vi "DPT TC Panel Setup.vi"() -> (6 "Channel List":string="1001,1002,1003", 8 "Label Array":string[](array[string])=["RDB F", "Room Ambient(F)", "Tscale"], 10 "Indexes used":i32[](array[numeric]))   [LabVIEW 2016]
doc: "Allow user to choose TCs to measure and save data for."
uses:
  Type Definitions/DPT Channel Label.ctl
  Utility/Custom Pallet Controls/Custom Pallet String.ctl
  <vilib>/Utility/file.llb/Read From Spreadsheet File (string).vi
  <vilib>/Utility/file.llb/Write To Spreadsheet File (string).vi
panel:
  out "all rows":string[][](array[string])
  out "error out":errorcluster={"status"=TRUE, "code"=1, "source"="Set Permissions in Panel DPT Channel Test Labels.vi<APPEND>\n<Not A Path>"}
  in  "TC Panel 4":T1[][](array[typedef])
  in  "Read":bool
  in  "Write":bool
  in  "Initialize":bool
  in  "Complete":bool
  in  "TC Panel 3":T1[][](array[typedef])
  in  "TC Panel 2":T1[][](array[typedef])
  in  "TC Panel 1":T1[][](array[typedef])=[[{"Label"="RDB F", "Record"=TRUE, "Index"=0, "Channel"=""}, {"Label"="Room Ambient(F)", "Record"=TRUE, "Index"=0, "Channel"=""}, {"Label"="Tscale", "Record"=TRUE, "Index"=0, "Channel"=""}, {"Label"="", "Record"=FALSE, "Index"=0, "Channel"=""}, {"Label"="", "Record"=FALSE, "Index"=0, "Channel"=""}, {"Label"="", "Record"=FALSE, "Index"=0, "Channel"=""}], [{"Label"="", "Record"=FALSE, "Index"=0, "Channel"=""}, {"Label"="", "Record"=FALSE, "Index"=0, "Channel"=""}, {"Label"="", "Record"=FALSE, "Index"=0, "Channel"=""}, {"Label"="", "Record"=FALSE, "Index"=0, "Channel"=""}, {"Label"="", "Record"=FALSE, "Index"=0, "Channel"=""}, {"Label"="", "Record"=FALSE, "Index"=0, "Channel"=""}], [{"Label"="", "Record"=FALSE, "Index"=0, "Channel"=""}, {"Label"="", "Record"=FALSE, "Index"=0, "Channel"=""}, {"Label"="", "Record"=FALSE, "Index"=0, "Channel"=""}, {"Label"="", "Record"=FALSE, "Index"=0, "Channel"=""}, {"Label"="", "Record"=FALSE, "Index"=0, "Channel"=""}, {"Label"="", "Record"=FALSE, "Index"=0, "Channel"=""}]]
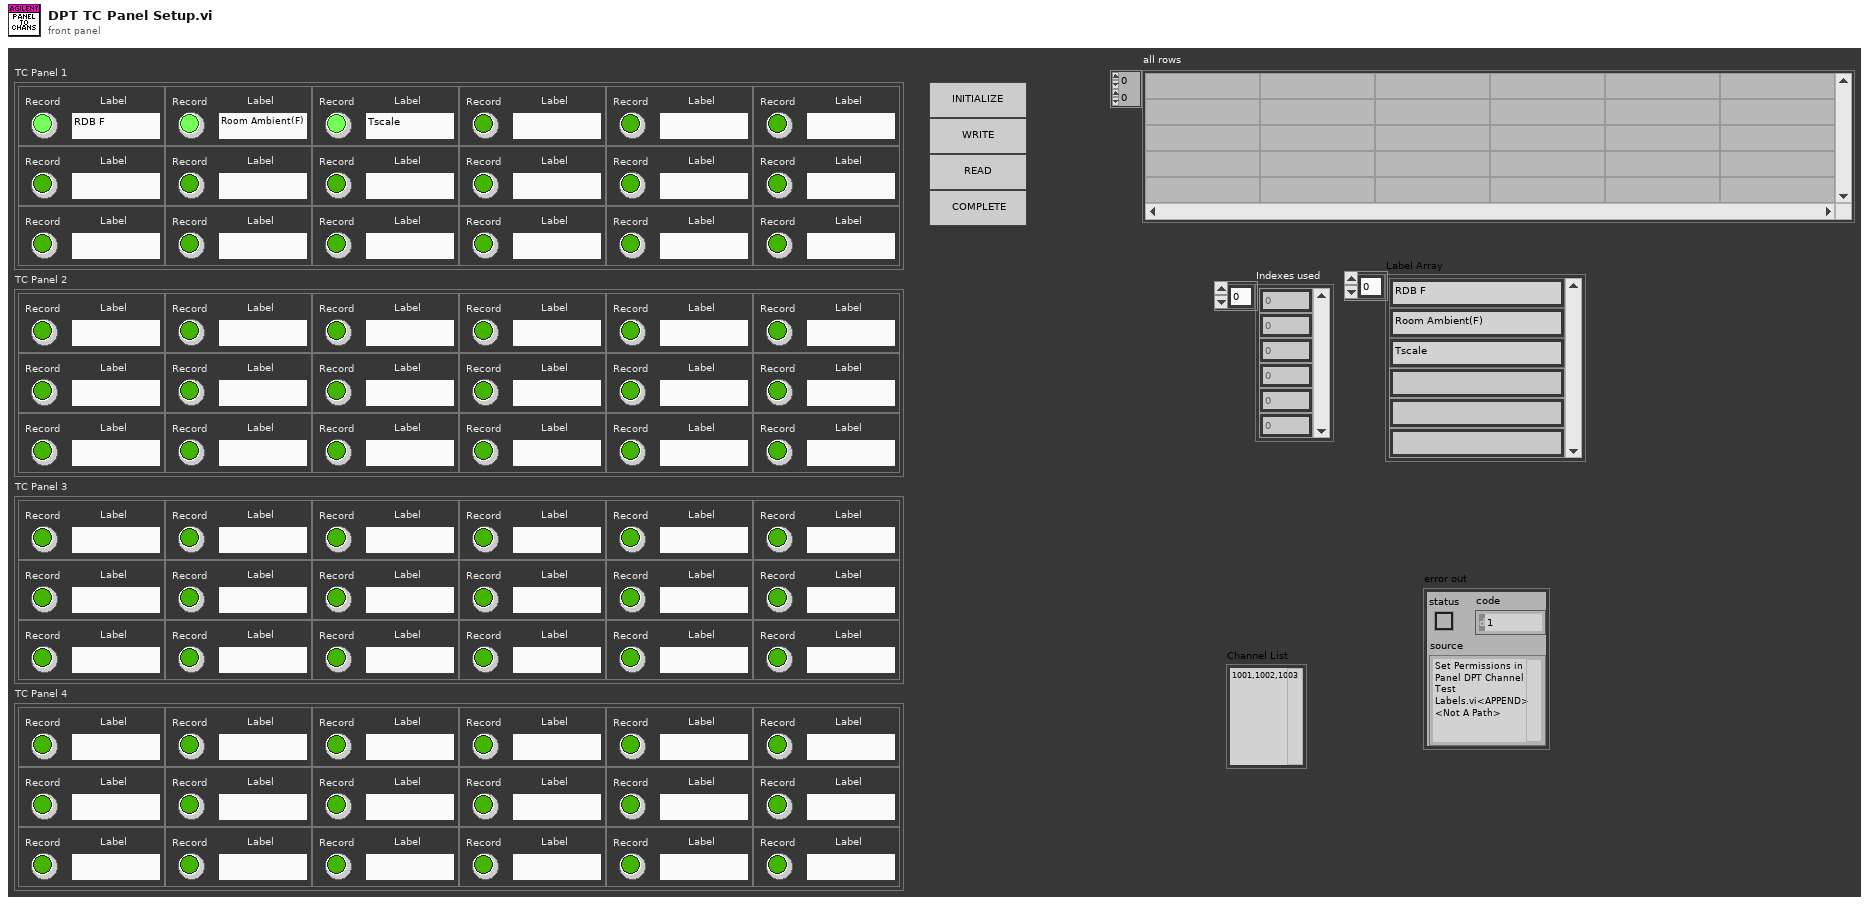
[diagram p1: front panel]
types:
  T1 = typedef "DPT Channel Label.ctl" = cluster{"Label":T2, "Record":bool, "Index":u32, "Channel":string}
  T2 = typedef "Custom Pallet String.ctl" = string
  T3 = enum32{"invalid app kind", "Development System", "Run Time System", "Student Edition", "Embedded LabVIEW", "Evaluation", "Custom"}
  T4 = enum32{"Invalid", "Standard", "Closed", "Hidden", "Minimized", "Maximized"}
  T5 = cluster{"Core":cluster{"Current VI Reference":refnum<vi>, "Close Panel on Exit?":bool}, "Array":string[][], "cDAQ index array":i32[][], "TC Panel 1":T1[][], "TC Panel 2":T1[][], "TC Panel 3":T1[][], "TC Panel 4":T1[][], "Label array":string[], "Channel array":string, "Indexes used":i32[]}
  T6 = cluster{"Current VI Reference":refnum<vi>, "Close Panel on Exit?":bool}
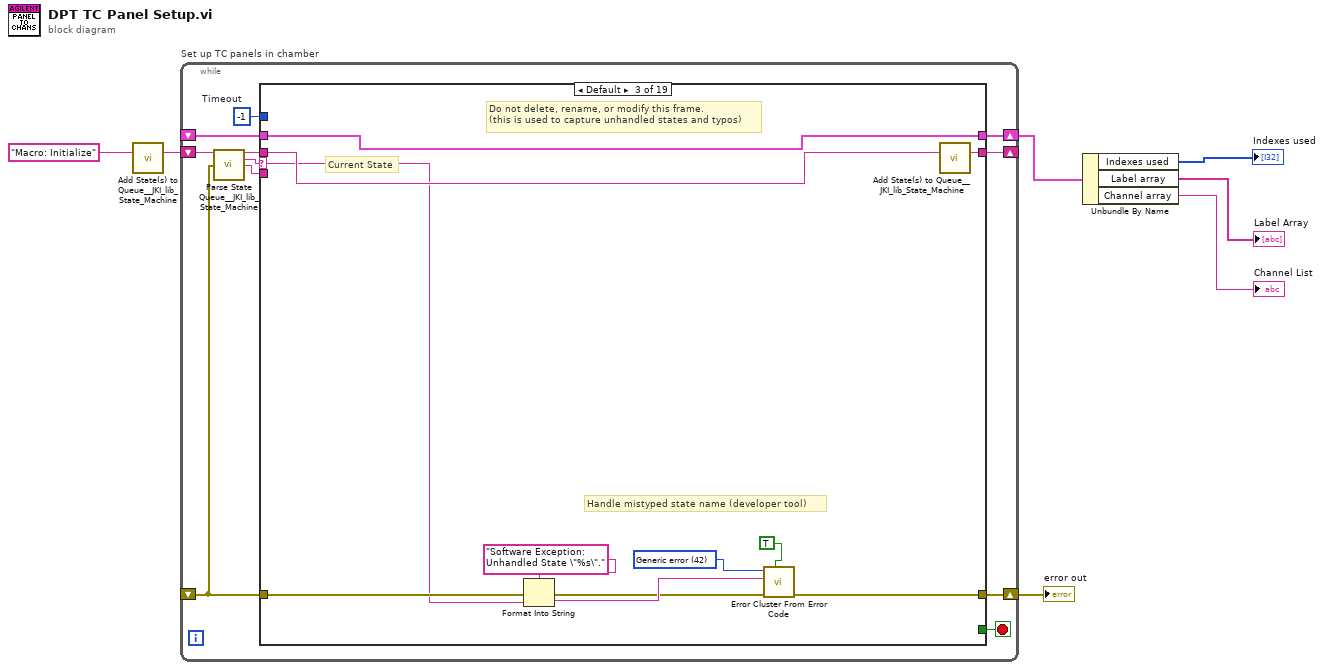
[diagram p0: block diagram]
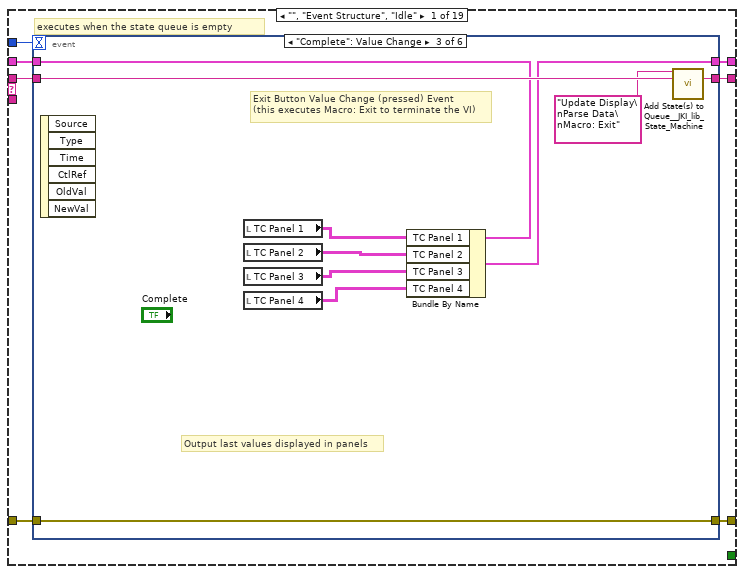
[diagram p2: hidden frame]
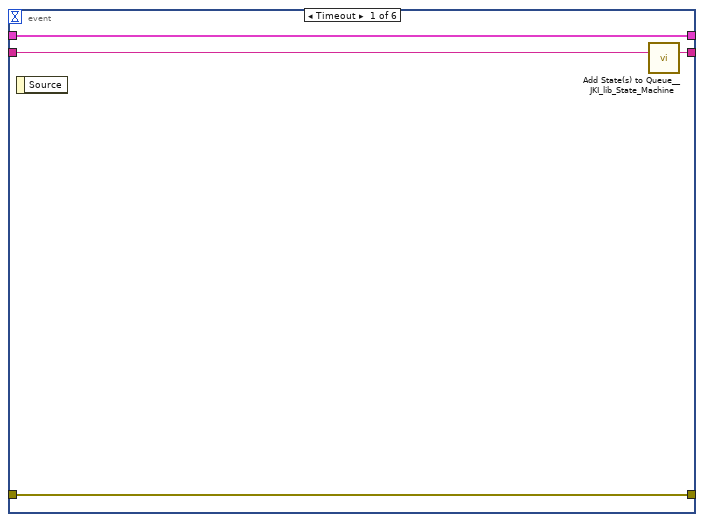
[diagram p3: hidden frame]
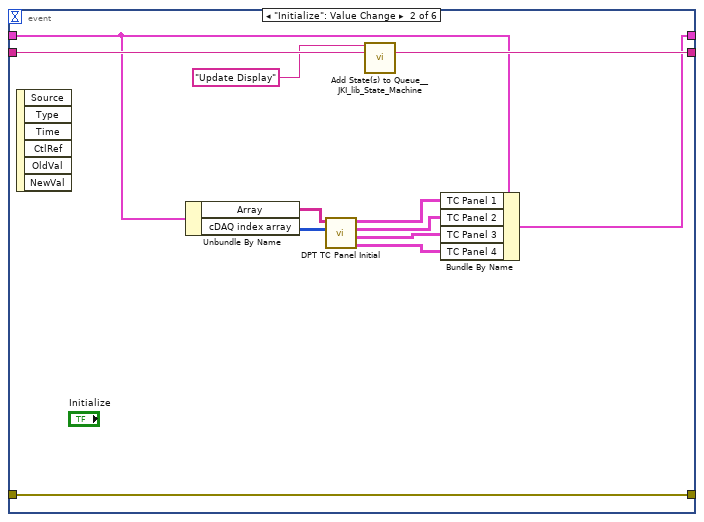
[diagram p4: hidden frame]
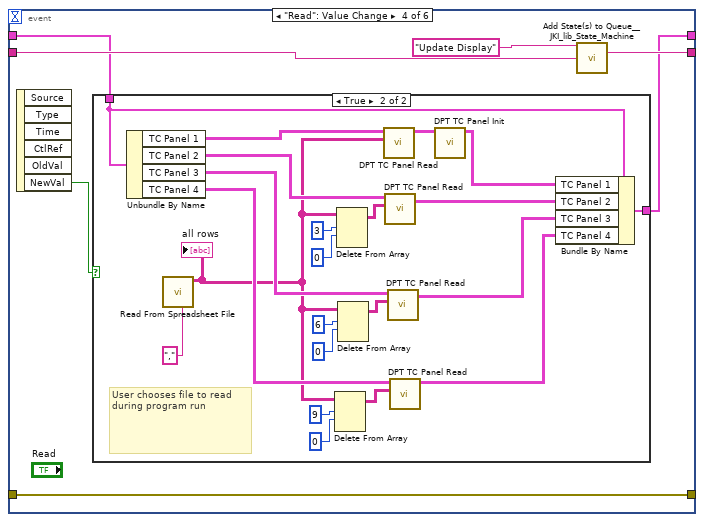
[diagram p5: hidden frame]
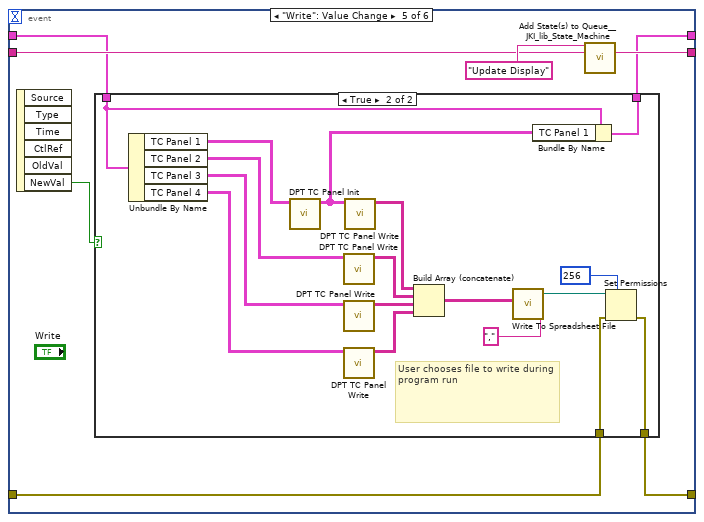
[diagram p7: hidden frame]
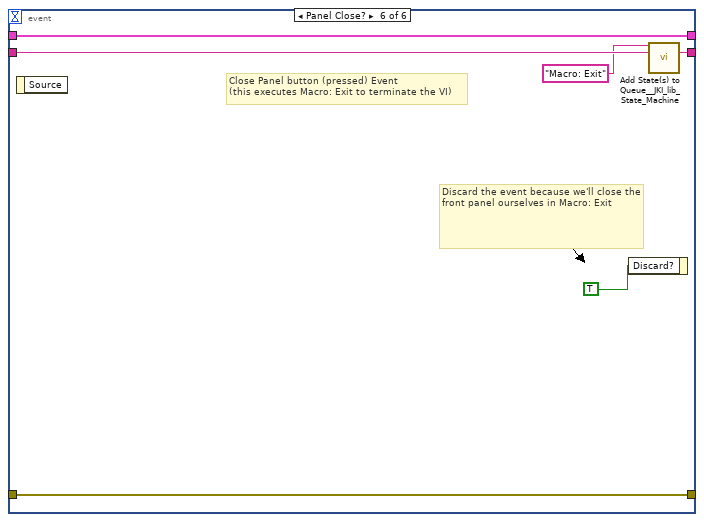
[diagram p9: hidden frame]
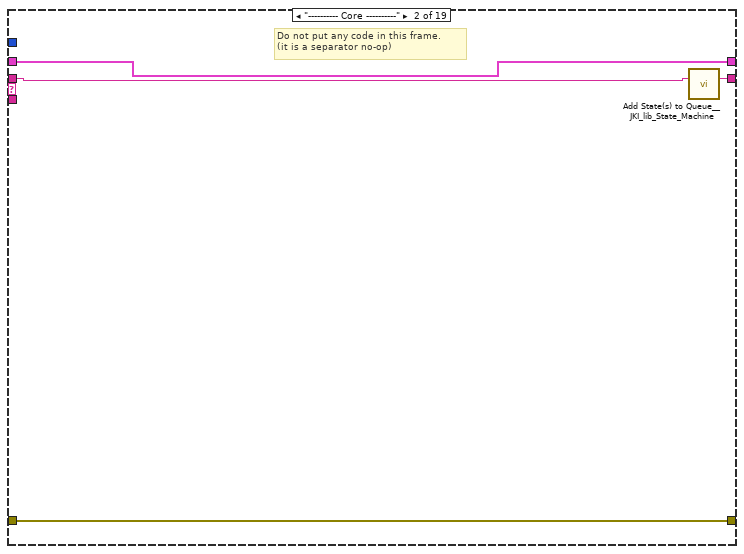
[diagram p10: hidden frame]
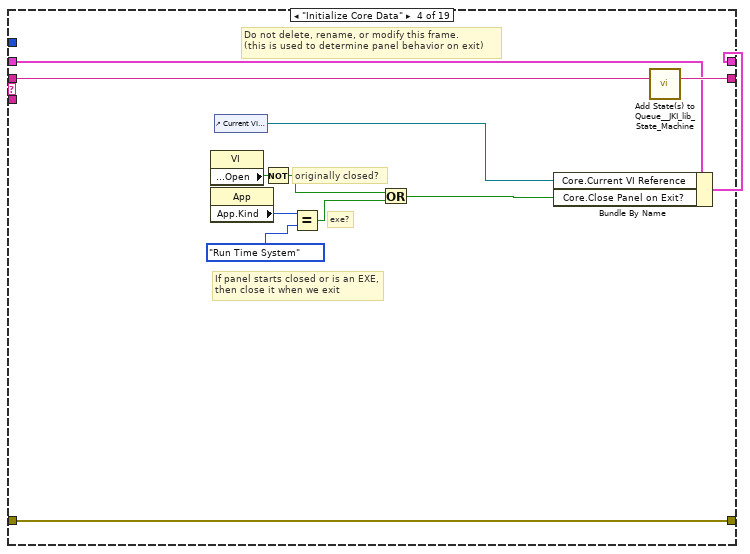
[diagram p11: hidden frame]
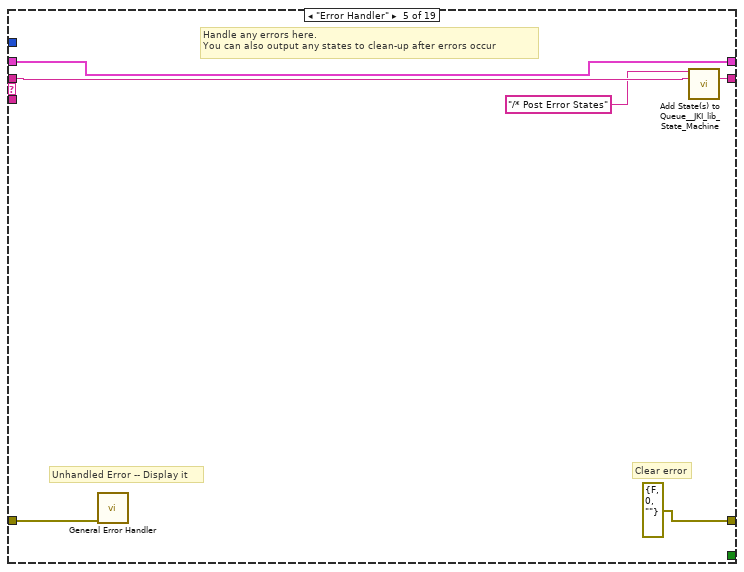
[diagram p12: hidden frame]
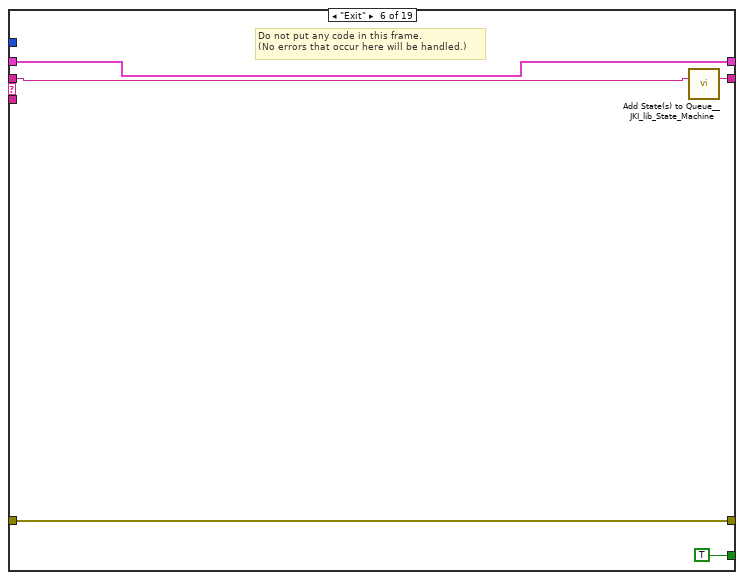
[diagram p13: hidden frame]
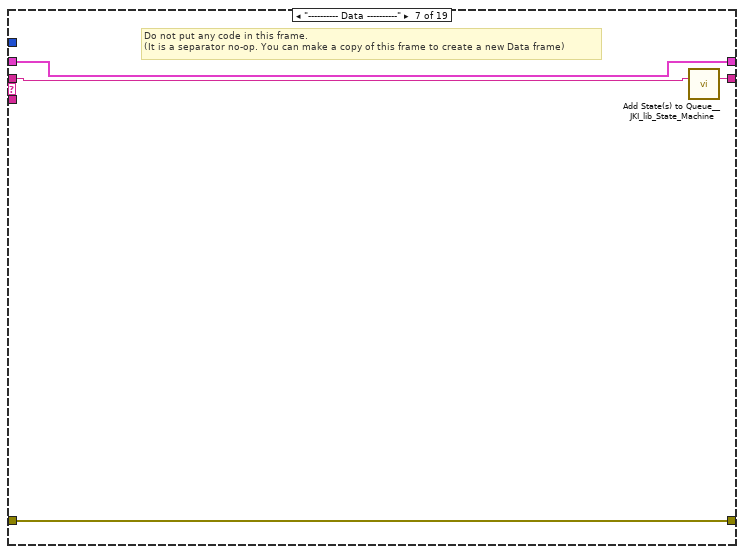
[diagram p14: hidden frame]
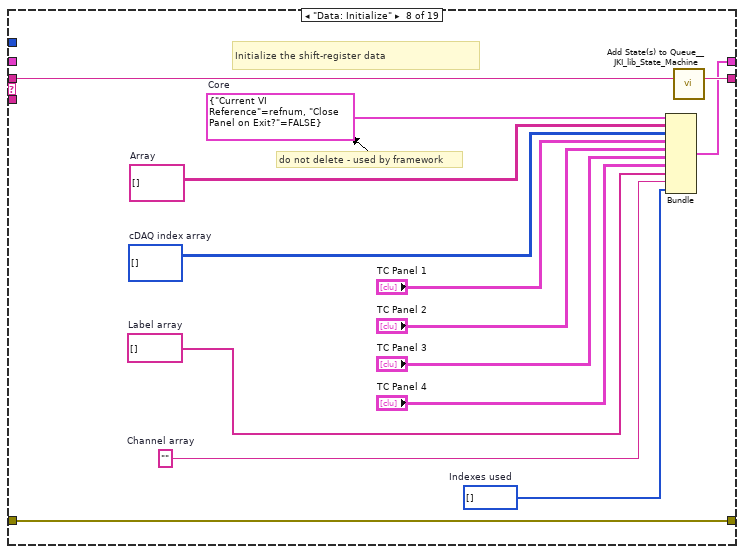
[diagram p15: hidden frame]
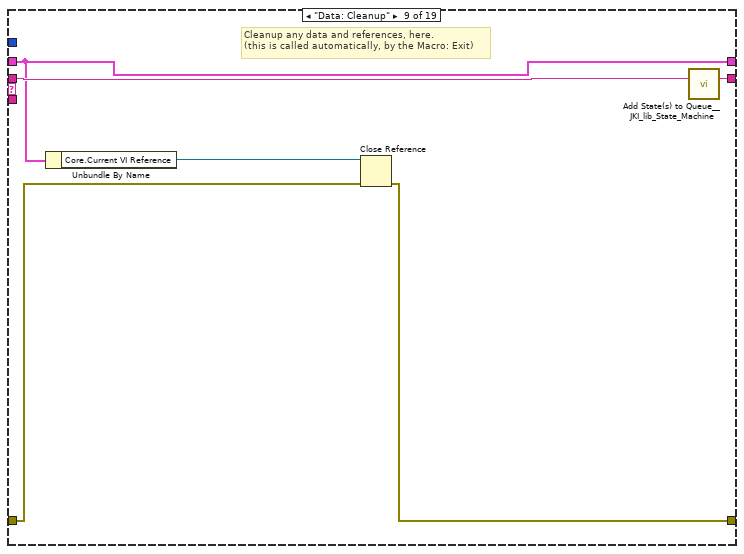
[diagram p16: hidden frame]
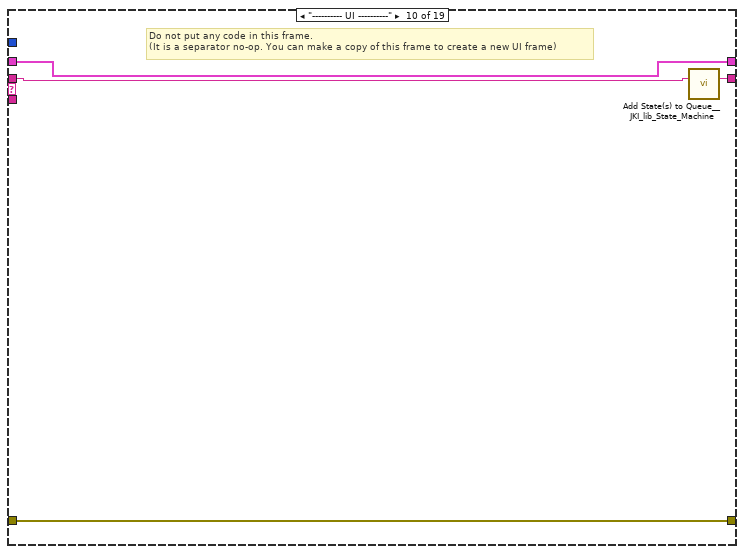
[diagram p17: hidden frame]
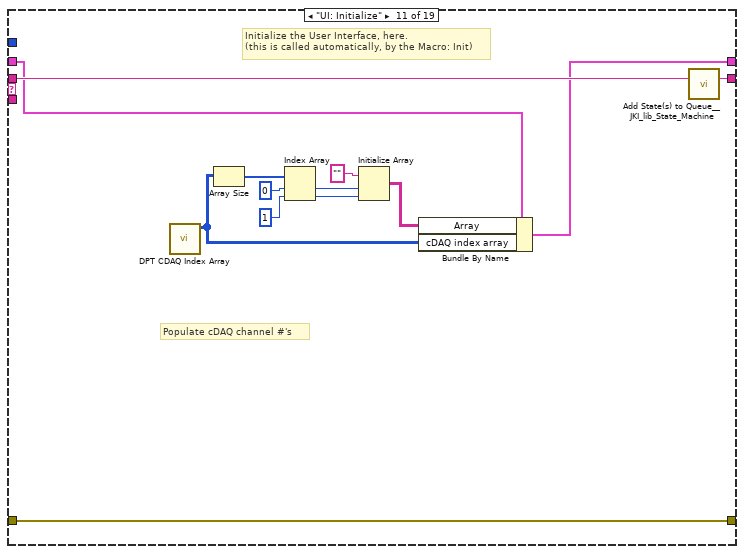
[diagram p18: hidden frame]
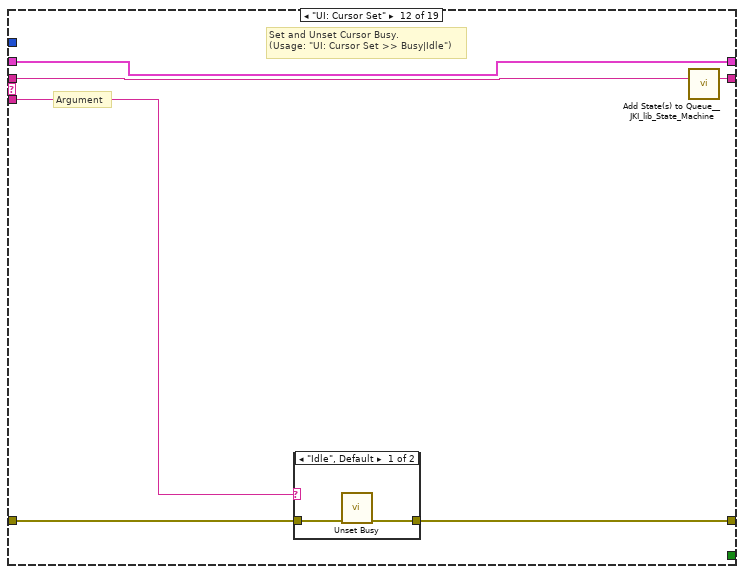
[diagram p19: hidden frame]
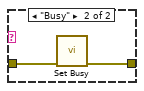
[diagram p20: hidden frame]
diagram:
  n1 = call <vilib>:"Add State(s) to Queue__JKI_lib_State_Machine.vi"("State(s) in (\"\")"="Macro: Initialize") -> ("States Out"=w7:string)  [unwired: 14 in]
  n2 = while "Set up TC panels in chamber" {
    shift-right: [w11] -> w5
    shift-left: _ -> [w10]
    shift-right: [w14] -> w4
    shift-left: _ -> [w8]
    shift-right: [w13] -> _
    shift-left: w7 -> [w15]
    stop <- w12 stop-if-true
    w9 = -1  # Timeout
    n3 = call <vilib>:"Parse State Queue__JKI_lib_State_Machine.vi"("State Queue"=w15, "Error In (no error)"=w8) -> ("Remaining States"=w17:string, "Current State"=w18:string, "Arguments"=w16:string)  [unwired: 11 in]
    n4 = case shown="Default" w18 {
      selector: w18 -> [_ _ w119 _ _ _ _ _ _ _ _ _ _ _ _ _ _ _ _]
      tunnel: w17 -> [w25 w118 w123 w141 w147 w152 w156 w170 w176 w180 w193 w199 w210 w236 w241 w251 w255 w263 w300]
      tunnel: w16 -> [_ _ _ _ _ _ _ _ _ _ _ w194 w204 _ _ _ _ _ _]
      tunnel: w10 -> [w23 w115 w121 w132 w144 w150 w153 _ w171 w177 w184 w197 w206 w233 w238 w248 w252 w260 w277]
      tunnel: [w22 w116 w125 w138 errorcluster {"status"=FALSE, "code"=0, "source"=""} ("error out") w149 w154 w167 w172 w178 w191 w195 w207 w234 w239 w249 w253 w261 w298] -> w14
      tunnel: w8 -> [w21 w116 w124 w138 w143 w149 w154 w167 w173 w178 w191 w196 w208 w234 w239 w249 w253 w261 w298]
      tunnel: [w24 w117 w122 w140 w146 w151 w155 w169 w175 w179 w192 w198 w209 w235 w240 w250 w254 w262 w299] -> w13
      tunnel: [_ _ _ _ _ TRUE _ _ _ _ _ _ _ _ _ _ _ _ _] -> w12
      tunnel: [w20 w115 w121 w139 w144 w150 w153 w168 w171 w177 w183 w197 w206 w233 w238 w248 w252 w260 w280] -> w11
      tunnel: w9 -> [w19 _ _ _ _ _ _ _ _ _ _ _ _ _ _ _ _ _ _]
      frame "", "Event Structure", "Idle" {
        # "executes when the state queue is empty"
        n5 = event shown="[2] \"Complete\": Value Change" {
          selector: _ -> [_ _ _ _ _ _]
          dyn-events: _ -> [_ _ _ _ _ _]
          timeout: w19 -> [_ _ _ _ _ _]
          tunnel: w25 -> [w29 w38 w51 w56 w86 w114]
          tunnel: [w28 w37 w50 w55 w85 w113] -> w24
          tunnel: w23 -> [w26 w35 w46 w54 w83 w111]
          tunnel: [w27 w41 w49 w58 w88 w112] -> w22
          tunnel: w21 -> [w27 w41 w49 w58 w89 w112]
          tunnel: [w26 w34 w47 w53 w84 w111] -> w20
          event Timeout {
            n6 = event-data() -> ()  [unwired: 1 in, 1 out]
            n7 = call <vilib>:"Add State(s) to Queue__JKI_lib_State_Machine.vi"("State(s) in (\"\")"=w29) -> ("States Out"=w28:string)  [unwired: 14 in]
          }
          event "Initialize": Value Change {
            n8 = event-data() -> ()  [unwired: 1 in, 6 out]
            n9 = Unbundle By Name(w35) -> ("Array"=w40:string[][], "cDAQ index array"=w39:i32[][])
            n10 = call "DPT TC Panel Initial.vi"("cDAQ index array"=w39, "Array"=w40) -> ("TC Panel 4"=w30:T1[][], "TC Panel 3"=w31:T1[][], "TC Panel 2"=w32:T1[][], "TC Panel 1"=w33:T1[][])  [unwired: 6 in]
            n11 = call <vilib>:"Add State(s) to Queue__JKI_lib_State_Machine.vi"("State(s) in Front (\"\")"="Update Display", "State(s) in (\"\")"=w38) -> ("States Out"=w37:string)  [unwired: 13 in]
            n12 = Bundle By Name(cluster=w35, "TC Panel 1"=w33, "TC Panel 2"=w32, "TC Panel 3"=w31, "TC Panel 4"=w30) -> (w34:T5)
          }
          event "Complete": Value Change {
            # "Output last values displayed in panels"
            # "Exit Button Value Change (pressed) Event\n(this executes Macro: Exit to terminate the VI)"
            n13 = event-data() -> ()  [unwired: 1 in, 6 out]
            n14 = local read "TC Panel 1"() -> (w45:T1[][])
            n15 = local read "TC Panel 2"() -> (w44:T1[][])
            n16 = local read "TC Panel 3"() -> (w43:T1[][])
            n17 = local read "TC Panel 4"() -> (w42:T1[][])
            n18 = Bundle By Name(cluster=w46, "TC Panel 1"=w45, "TC Panel 2"=w44, "TC Panel 3"=w43, "TC Panel 4"=w42) -> (w47:T5)
            n19 = call <vilib>:"Add State(s) to Queue__JKI_lib_State_Machine.vi"("State(s) in Front (\"\")"="Update Display\nParse Data\nMacro: Exit", "State(s) in (\"\")"=w51) -> ("States Out"=w50:string)  [unwired: 13 in]
          }
          event "Read": Value Change {
            n20 = event-data() -> ("NewVal"=w52:bool)  [unwired: 1 in, 5 out]
            n21 = case shown="True" w52 {
              tunnel: w54 -> [w59 w68]
              tunnel: [w59 w67] -> w53
              frame False {
              }
              frame True {
                # "User chooses file to read during program run"
                n22 = Unbundle By Name(w68) -> ("TC Panel 1"=w73:T1[][], "TC Panel 2"=w72:T1[][], "TC Panel 3"=w71:T1[][], "TC Panel 4"=w70:T1[][])
                n23 = call-poly <vilib>:"Read From Spreadsheet File.vi"("delimiter (\\t)"="," ("delimiter (\\t)")) -> ("all rows"=w69:string[][])  [unwired: 6 in, 4 out]
                "all rows" <- w69
                n24 = Delete From Array(array=w69, length=9, index (row)=0) -> (array with subset deleted=w63:string[][])  [unwired: 1 in, 1 out]
                n25 = Delete From Array(array=w69, length=3, index (row)=0) -> (array with subset deleted=w81:string[][])  [unwired: 1 in, 1 out]
                n26 = Delete From Array(array=w69, length=6, index (row)=0) -> (array with subset deleted=w80:string[][])  [unwired: 1 in, 1 out]
                n27 = call "DPT TC Panel Read.vi"("all rows"=w69, "TC Panel 1"=w73) -> ("TC Panel 2"=w61:T1[][])  [unwired: 9 in]
                n28 = call "DPT TC Panel Read.vi"("all rows"=w81, "TC Panel 1"=w72) -> ("TC Panel 2"=w66:T1[][])  [unwired: 9 in]
                n29 = call "DPT TC Panel Read.vi"("all rows"=w80, "TC Panel 1"=w71) -> ("TC Panel 2"=w65:T1[][])  [unwired: 9 in]
                n30 = call "DPT TC Panel Read.vi"("all rows"=w63, "TC Panel 1"=w70) -> ("TC Panel 2"=w64:T1[][])  [unwired: 9 in]
                n31 = call "DPT TC Panel Init.vi"("TC Panel"=w61) -> ("TC Panel 1"=w60:T1[][])  [unwired: 10 in]
                n32 = Bundle By Name(cluster=w68, "TC Panel 1"=w60, "TC Panel 2"=w66, "TC Panel 3"=w65, "TC Panel 4"=w64) -> (w67:T5)
              }
            }
            n33 = call <vilib>:"Add State(s) to Queue__JKI_lib_State_Machine.vi"("State(s) in Front (\"\")"="Update Display", "State(s) at Back (\"\")"=w56) -> ("States Out"=w55:string)  [unwired: 13 in]
          }
          event "Write": Value Change {
            n34 = event-data() -> ("NewVal"=w82:bool)  [unwired: 1 in, 5 out]
            n35 = case shown="True" w82 {
              tunnel: w89 -> [w91 w100]
              tunnel: [w91 w99] -> w88
              tunnel: [w90 w95] -> w84
              tunnel: w83 -> [w90 w94]
              frame False {
              }
              frame True {
                # "User chooses file to write during program run"
                n36 = Unbundle By Name(w94) -> ("TC Panel 1"=w93:T1[][], "TC Panel 2"=w98:T1[][], "TC Panel 3"=w97:T1[][], "TC Panel 4"=w96:T1[][])
                n37 = call "DPT TC Panel Init.vi"("TC Panel"=w93) -> ("TC Panel 1"=w92:T1[][])  [unwired: 10 in]
                n38 = call "DPT TC Panel Write.vi"("TC Panel 1 Out"=w98) -> ("Array"=w107:string[][])  [unwired: 10 in]
                n39 = call "DPT TC Panel Write.vi"("TC Panel 1 Out"=w97) -> ("Array"=w108:string[][])  [unwired: 10 in]
                n40 = call "DPT TC Panel Write.vi"("TC Panel 1 Out"=w96) -> ("Array"=w106:string[][])  [unwired: 10 in]
                n41 = call "DPT TC Panel Write.vi"("TC Panel 1 Out"=w92) -> ("Array"=w105:string[][])  [unwired: 10 in]
                n42 = Build Array (concatenate)(w105, w107, w108, w106) -> (w103:string[][])
                n43 = call-poly <vilib>:"Write To Spreadsheet File.vi"("delimiter (\\t)"="," ("delimiter (\\t)"), "2D data"=w103) -> ("new file path (Not A Path if cancelled)"=w104:path)  [unwired: 6 in]
                n44 = Bundle By Name(cluster=w94, "TC Panel 1"=w92) -> (w95:T5)
                n45 = Set Permissions(7:i16 256 ("permissions"), 8:w100, 11:w104) -> (0:w99:errorcluster)  [unwired: 2 in, 1 out]
              }
            }
            n46 = call <vilib>:"Add State(s) to Queue__JKI_lib_State_Machine.vi"("State(s) in Front (\"\")"="Update Display", "State(s) in (\"\")"=w86) -> ("States Out"=w85:string)  [unwired: 13 in]
          }
          event Panel Close? {
            # "Discard the event because we'll close the front panel ourselves in Macro: Exit"
            # "Close Panel button (pressed) Event\n(this executes Macro: Exit to terminate the VI)"
            n47 = event-data() -> ()  [unwired: 1 in, 1 out]
            n48 = event-data("Discard?"=TRUE) -> ()  [unwired: 1 in, 1 out]
            n49 = call <vilib>:"Add State(s) to Queue__JKI_lib_State_Machine.vi"("State(s) in Front (\"\")"="Macro: Exit", "State(s) in (\"\")"=w114) -> ("States Out"=w113:string)  [unwired: 13 in]
          }
        }
      }
      frame "---------- Core ----------" {
        # "Do not put any code in this frame.\n(it is a separator no-op)"
        n50 = call <vilib>:"Add State(s) to Queue__JKI_lib_State_Machine.vi"("State(s) in (\"\")"=w118) -> ("States Out"=w117:string)  [unwired: 14 in]
      }
      frame Default {
        w128 = 42 items=["No error", "Argument error", "Memory is full", "Out of zone", "End of file", "File already open", "Generic file I/O error", "File not found", "File permission error", "Disk is full", "Duplicate path", "Too many files open", "System feature not enabled", "Resource file not found", "Cannot add resource", "Resource not found", "Image not found", "Image memory error", "Pen does not exist", "Config type invalid", "Config token not found", "Config parse error", "Config memory error", "Bad external code format", "Bad external code offset", "External code not present", "Null window", "Destroy window error", "Null menu", "Print aborted", "Bad print record", "Print driver error", "Windows error during printing", "Memory error during printing", "Print dialog error", "Generic print error", "Invalid device refnum", "Device not found", "Device parameter error", "Device unit error", "Cannot open device", "Device call aborted", "Generic error", "Cancelled by user", "Object ID too low", "Object ID too high", "Object not in heap", "Unknown heap", "Unknown object (invalid DefProc)", "Unknown object (DefProc not in table)", "Message out of range", "Invalid (null) method", "Unknown message", "Manager call not supported", "Bad address", "Network operation in progress", "Network operation timed out", "Connection is busy", "Network attribute not supported", "Network error", "Address in use", "System out of memory", "Connection aborted", "Connection refused", "Not connected", "Already connected", "Connection closed", "Initialization error (interapplication manager)", "Bad occurrence", "Wait on unbound occurrence handler", "Occurrence queue overflow", "Datalog type conflict", "Unused", "Unrecognized type (interapplication manager)", "Memory corrupt", "Failed to make temporary DLL", "Old CIN version", "Drag socket not found", "Failed to load drop-object", "Failed to register OLE object", "Failed to release OLE object", "Format specifier type mismatch", "Unknown format specifier", "Too few format specifiers", "Too many format specifiers", "Scan failed", "Newer CIN version", "Error converting to variant", "Runtime menu error", "Password tampered", "Variant attribute not found", "Incompatible variant data type", "Event data is not available", "Event Store is not present", "Occurrence is not found", "Event Queue is not created", "Event info is not available", "Refnum passed is NULL", "Error retrieving Class GUID", "Error retrieving CoClass GUID", "Error retrieving TypeLib GUID.", "Bad built application magic bytes.", "Specific driver is different from the specific driver associated with the Logical Name.", "There is no session opened to the class driver.", "Max Error", "MAX - Error with config objects", "MAX - Error loading configuration", "MAX - Group not supported"]
        # "Current State"
        # "Do not delete, rename, or modify this frame.\n(this is used to capture unhandled states and typos)"
        # "Handle mistyped state name (developer tool)"
        n51 = Format Into String(format string="Software Exception: Unhandled State \"%s\"." ("message"), error in=w124, w119) -> (resulting string=w127:string, error out=w126:errorcluster)  [unwired: 1 in]
        n52 = call <vilib>:"Error Cluster From Error Code.vi"("show call chain? (False)"=TRUE, "error in (no error)"=w126, "error message (\"\")"=w127, "error code (0)"=w128) -> ("error out"=w125:errorcluster)  [unwired: 5 in]
        n53 = call <vilib>:"Add State(s) to Queue__JKI_lib_State_Machine.vi"("State(s) in (\"\")"=w123) -> ("States Out"=w122:string)  [unwired: 14 in]
      }
      frame "Initialize Core Data" {
        # "Do not delete, rename, or modify this frame.\n(this is used to determine panel behavior on exit)"
        # "originally closed?"
        # "exe?"
        # "If panel starts closed or is an EXE, then close it when we exit"
        n54 = property class="VI"() -> ("Front Panel.Open"=w137:bool)  [unwired: 2 in, 2 out]
        n55 = property class="App"() -> ("App.Kind"=w136:T3)  [unwired: 2 in, 2 out]
        n56 = control-ref of="Current VI Reference"() -> (w130:refnum<vi>)
        n57 = Not(x=w137) -> (.not. x?=w134:bool)
        n58 = Equal?(x=w136, y=T3."Run Time System" ("Application:Kind")) -> (x = y?=w133:bool)
        n59 = Or(x=w134, y=w133) -> (x .or. y?=w131:bool)
        n60 = Bundle By Name(cluster=w132, "Core.Current VI Reference"=w130, "Core.Close Panel on Exit?"=w131) -> (w139:T5)
        n61 = call <vilib>:"Add State(s) to Queue__JKI_lib_State_Machine.vi"("State(s) in (\"\")"=w141) -> ("States Out"=w140:string)  [unwired: 14 in]
      }
      frame "Error Handler" {
        # "Unhandled Error -- Display it"
        # "Handle any errors here.\nYou can also output any states to clean-up after errors occur"
        # "Clear error"
        n62 = call <vilib>:"General Error Handler.vi"("error in (no error)"=w143) -> ()  [unwired: 10 in, 5 out]
        n63 = call <vilib>:"Add State(s) to Queue__JKI_lib_State_Machine.vi"("State(s) in Front (\"\")"="/* Post Error States", "State(s) in (\"\")"=w147) -> ("States Out"=w146:string)  [unwired: 13 in]
      }
      frame "Exit" {
        # "Do not put any code in this frame.\n(No errors that occur here will be handled.)"
        n64 = call <vilib>:"Add State(s) to Queue__JKI_lib_State_Machine.vi"("State(s) in (\"\")"=w152) -> ("States Out"=w151:string)  [unwired: 14 in]
      }
      frame "---------- Data ----------" {
        # "Do not put any code in this frame.\n(It is a separator no-op. You can make a copy of this frame to create a new Data frame)"
        n65 = call <vilib>:"Add State(s) to Queue__JKI_lib_State_Machine.vi"("State(s) in (\"\")"=w156) -> ("States Out"=w155:string)  [unwired: 14 in]
      }
      frame "Data: Initialize" {
        w157 = string[] []  # Label array
        w158 = i32[] []  # Indexes used
        w159 = ""  # Channel array
        w164 = i32[][] []  # cDAQ index array
        w165 = string[][] []  # Array
        w166 = T6 {"Current VI Reference"=refnum, "Close Panel on Exit?"=FALSE}  # Core
        # "do not delete - used by framework"
        # "Initialize the shift-register data"
        n66 = Bundle("Core"=w166, "Array"=w165, "cDAQ index array"=w164, "TC Panel 1"="TC Panel 1", "TC Panel 2"="TC Panel 2", "TC Panel 3"="TC Panel 3", "TC Panel 4"="TC Panel 4", "Label array"=w157, "Channel array"=w159, "Indexes used"=w158) -> (w168:T5)  [unwired: 1 in]
        n67 = call <vilib>:"Add State(s) to Queue__JKI_lib_State_Machine.vi"("State(s) in (\"\")"=w170) -> ("States Out"=w169:string)  [unwired: 14 in]
      }
      frame "Data: Cleanup" {
        # "Cleanup any data and references, here.\n(this is called automatically, by the Macro: Exit)"
        n68 = Unbundle By Name(w171) -> ("Core.Current VI Reference"=w174:refnum<vi>)
        n69 = Close Reference(reference=w174, error in (no error)=w173) -> (error out=w172:errorcluster)
        n70 = call <vilib>:"Add State(s) to Queue__JKI_lib_State_Machine.vi"("State(s) in (\"\")"=w176) -> ("States Out"=w175:string)  [unwired: 14 in]
      }
      frame "---------- UI ----------" {
        # "Do not put any code in this frame.\n(It is a separator no-op. You can make a copy of this frame to create a new UI frame)"
        n71 = call <vilib>:"Add State(s) to Queue__JKI_lib_State_Machine.vi"("State(s) in (\"\")"=w180) -> ("States Out"=w179:string)  [unwired: 14 in]
      }
      frame "UI: Initialize" {
        # "Populate cDAQ channel #'s"
        # "Initialize the User Interface, here.\n(this is called automatically, by the Macro: Init)"
        n72 = call "DPT CDAQ Index Array.vi"() -> ("cDAQ Index"=w181:i32[][])  [unwired: 9 in, 1 out]
        n73 = Array Size(array=w181) -> (size(s)=w185:i32[])
        n74 = Index Array(array=w185, index #1=0 ("index"), index #2=1 ("index")) -> (element #1=w188:i32, element #2=w189:i32)
        n75 = Initialize Array("", w188, w189) -> (w182:string[][])
        n76 = Bundle By Name(cluster=w184, "Array"=w182, "cDAQ index array"=w181) -> (w183:T5)
        n77 = call <vilib>:"Add State(s) to Queue__JKI_lib_State_Machine.vi"("State(s) in (\"\")"=w193) -> ("States Out"=w192:string)  [unwired: 14 in]
      }
      frame "UI: Cursor Set" {
        # "Argument"
        # "Set and Unset Cursor Busy.\n(Usage: \"UI: Cursor Set >> Busy|Idle\")"
        n78 = case shown="\"Idle\", Default" w194 {
          tunnel: w196 -> [w201 w203]
          tunnel: [w200 w202] -> w195
          frame "Idle", Default {
            n79 = call <vilib>:"Unset Busy.vi"("error in (no error)"=w201) -> ("error out"=w200:errorcluster)  [unwired: 10 in]
          }
          frame "Busy" {
            n80 = call <vilib>:"Set Busy.vi"("error in (no error)"=w203) -> ("error out"=w202:errorcluster)  [unwired: 9 in, 1 out]
          }
        }
        n81 = call <vilib>:"Add State(s) to Queue__JKI_lib_State_Machine.vi"("State(s) in (\"\")"=w199) -> ("States Out"=w198:string)  [unwired: 14 in]
      }
      frame "UI: Front Panel State" {
        # "Argument"
        # "Set Front Panel Open or Closed\n(Usage: \"UI: Front Panel State >> Open|Close\")"
        n82 = Unbundle By Name(w206) -> ("Core.Current VI Reference"=w205:refnum<vi>)
        n83 = case shown="\"Open\", Default" w204 {
          tunnel: w208 -> [w214 w227]
          tunnel: [w216 w228] -> w207
          tunnel: w205 -> [w215 w225]
          frame "Open", Default {
            n84 = property class="VI"(reference=w215, error in=w214) -> (reference out=w212:refnum<vi>, error out=w213:errorcluster, "Front Panel.Open"=w211:bool)
            n85 = case shown="True" w211 {
              tunnel: [w219 w222] -> w216
              tunnel: w213 -> [w218 w222]
              tunnel: w212 -> [w217 _]
              frame False {
                n86 = invoke class="VI" method="FP.Open"(reference=w217, error in=w218, "Activate"=TRUE, "State"=T4."Standard") -> (error out=w219:errorcluster)  [unwired: 1 in, 4 out]
              }
              frame True {
              }
            }
          }
          frame "Close" {
            n87 = property class="VI"(reference=w225, error in=w227) -> (reference out=w224:refnum<vi>, error out=w226:errorcluster, "Front Panel.Open"=w223:bool)
            n88 = case shown="True" w223 {
              tunnel: [w229 w232] -> w228
              tunnel: w226 -> [w229 w231]
              tunnel: w224 -> [_ w230]
              frame False {
              }
              frame True {
                n89 = invoke class="VI" method="FP.Close"(reference=w230, error in=w231) -> (error out=w232:errorcluster)  [unwired: 1 in, 2 out]
              }
            }
          }
        }
        n90 = call <vilib>:"Add State(s) to Queue__JKI_lib_State_Machine.vi"("State(s) in (\"\")"=w210) -> ("States Out"=w209:string)  [unwired: 14 in]
      }
      frame "---------- Macro ----------" {
        # "Do not put any code in this frame.\n(It is a separator no-op. You can make a copy of this frame to create a new Macro frame)"
        n91 = call <vilib>:"Add State(s) to Queue__JKI_lib_State_Machine.vi"("State(s) in (\"\")"=w236) -> ("States Out"=w235:string)  [unwired: 14 in]
      }
      frame "Macro: Initialize" {
        w237 = "Data: Initialize\nInitialize Core Data\nUI: Initialize\nUI: Front Panel State >> Open"  # Data: Initialize Initialize Core Data UI: Initialize UI: Front Panel State >> Open
        n92 = call <vilib>:"Add State(s) to Queue__JKI_lib_State_Machine.vi"("State(s) in Front (\"\")"=w237, "State(s) in (\"\")"=w241) -> ("States Out"=w240:string)  [unwired: 13 in]
      }
      frame "Macro: Exit" {
        # "Exit Macro\n(This is called once, when the VI exits)"
        n93 = Unbundle By Name(w248) -> ("Core.Close Panel on Exit?"=w247:bool)
        n94 = Select(t="UI: Front Panel State >> Close", s=w247, f="") -> (s? t:f=w244:string)
        n95 = call <vilib>:"Add State(s) to Queue__JKI_lib_State_Machine.vi"("State(s) in (\"\")"=w244, "State(s) at Back (\"\")"="Data: Cleanup\nExit") -> ("States Out"=w242:string)  [unwired: 13 in]
        n96 = call <vilib>:"Add State(s) to Queue__JKI_lib_State_Machine.vi"("State(s) in Front (\"\")"=w242, "State(s) in (\"\")"=w251) -> ("States Out"=w250:string)  [unwired: 13 in]
      }
      frame "---------- New Category ----------" {
        # "Template Separator\n(You can make a copy of, or modify, this frame)"
        n97 = call <vilib>:"Add State(s) to Queue__JKI_lib_State_Machine.vi"("State(s) in (\"\")"=w255) -> ("States Out"=w254:string)  [unwired: 14 in]
      }
      frame "Update Display" {
        # "Update TC panel controls"
        n98 = Unbundle By Name(w260) -> ("TC Panel 1"=w259:T1[][], "TC Panel 2"=w258:T1[][], "TC Panel 3"=w257:T1[][], "TC Panel 4"=w256:T1[][])
        n99 = local write "TC Panel 1"(w259) -> ()
        n100 = local write "TC Panel 2"(w258) -> ()
        n101 = local write "TC Panel 3"(w257) -> ()
        n102 = local write "TC Panel 4"(w256) -> ()
        n103 = call <vilib>:"Add State(s) to Queue__JKI_lib_State_Machine.vi"("State(s) in (\"\")"=w263) -> ("States Out"=w262:string)  [unwired: 14 in]
      }
      frame "Parse Data" {
        # "Make channel list: 1001, 1002, 1003, etc."
        # "Panel #"
        # "Analyze data from TC panel controls: Panel location, label name, channel number\nCurrently, channel # is left blank (done inside Panel Parser.vi)"
        n104 = Unbundle By Name(w277) -> ("TC Panel 1"=w276:T1[][], "TC Panel 2"=w275:T1[][], "TC Panel 3"=w274:T1[][], "TC Panel 4"=w273:T1[][])
        n105 = call "DPT TC Panel Parser.vi"("Index start"=0, "Panel Num"="1-" ("String"), "TC Panel 1"=w276) -> ("Indexes Used"=w268:i32[], "Channel Array"=w287:string[], "Label Array"=w286:T2[])  [unwired: 6 in]
        n106 = call "DPT TC Panel Parser.vi"("Index start"=18, "Panel Num"="2-" ("String"), "TC Panel 1"=w275) -> ("Indexes Used"=w267:i32[], "Channel Array"=w291:string[], "Label Array"=w290:T2[])  [unwired: 6 in]
        n107 = call "DPT TC Panel Parser.vi"("Index start"=36, "Panel Num"="3-" ("String"), "TC Panel 1"=w274) -> ("Indexes Used"=w266:i32[], "Channel Array"=w294:string[], "Label Array"=w293:T2[])  [unwired: 6 in]
        n108 = call "DPT TC Panel Parser.vi"("Index start"=54, "Panel Num"="4-" ("String"), "TC Panel 1"=w273) -> ("Indexes Used"=w265:i32[], "Channel Array"=w297:string[], "Label Array"=w296:T2[])  [unwired: 6 in]
        n109 = Build Array (concatenate)(w286, w290, w293, w296) -> (w278:T2[])
        n110 = Build Array (concatenate)(w287, w291, w294, w297) -> (w281:string[])
        n111 = Build Array (concatenate)(w268, w267, w266, w265) -> (w264:i32[])
        n112 = for {
          tunnel: w281 -> [w303] mode=indexing
          shift-right: [w302] -> w283
          shift-left: "" -> [w301]
          n113 = Concatenate Strings(w301, w303, "," ("string")) -> (w302:string)
        }
        n114 = String Length(string=w283) -> (length=w285:i32)
        n115 = Decrement(x=w285) -> (x-1=w284:i32)
        n116 = String Subset(string=w283, length (rest)=w284) -> (substring=w279:string)  [unwired: 1 in]
        n117 = Bundle By Name(cluster=w277, "Label array"=w278, "Channel array"=w279, "Indexes used"=w264) -> (w280:T5)
        n118 = call <vilib>:"Add State(s) to Queue__jki_lib_state_machine.vi"("State(s) in (\"\")"=w300) -> ("States Out"=w299:string)  [unwired: 14 in]
      }
    }
  }
  "error out" <- w4
  n119 = Unbundle By Name(w5) -> ("Indexes used"=→"Indexes used":i32[], "Label array"=→"Label Array":string[], "Channel array"=→"Channel List":string)
